vi "Execute Message Async.vi"(8 "error in (no error)":errorcluster, 11 "Consumer":refnum<class "Abstract Consumer.lvclass">) -> (0 "error out":errorcluster)   [LabVIEW 2027, in "Multi Consumer Test Case.lvclass"]
uses:
  Multi Consumer Test Case.lvclass
  Consumer/Abstract Consumer/Abstract Consumer.lvclass
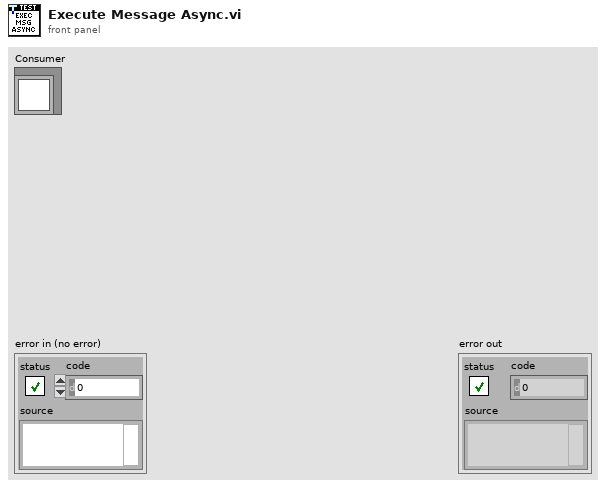
[diagram p1: front panel]
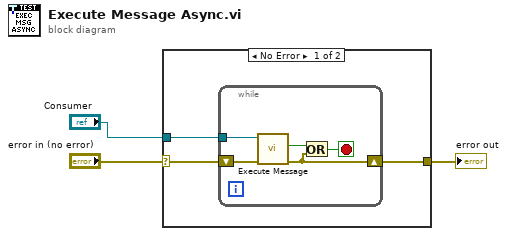
[diagram p0: block diagram]
diagram:
  n1 = case shown="No Error" "error in (no error)" {
    selector: "error in (no error)" -> [w6 w12]
    tunnel: [w5 w12] -> w2
    tunnel: "Consumer" -> [w4 _]
    frame No Error {
      n2 = while {
        shift-right: [w9] -> w5
        shift-left: w6 -> [w11]
        tunnel: w4 -> [w7]
        stop <- w8 stop-if-true
        n3 = call "Execute Message.vi"("error in (no error)"=w11, "Abstract Consumer in"=w7) -> ("error out"=w9:errorcluster, "Stop?"=w10:bool)  [unwired: 6 in, 2 out]
        n4 = Or(x=w10, y=w9) -> (x .or. y?=w8:bool)
      }
    }
    frame Error {
    }
  }
  "error out" <- w2
